vi "llh2lcctmp.vi"(7 "map name":T1(ring)=enum."KAIST", 9 "hgt[deg]":i32, 10 "lon[deg]":dbl format="%#_12f", 11 "lat[deg]":dbl format="%#_12f") -> (3 "LCC[m]":dbl[](array[numeric]))   [LabVIEW 2015]
uses:
  <vilib>/Analysis/Matrix/Numeric/Conversions/Array To Matrix - RA2.vi
  <vilib>/Analysis/Matrix/Numeric/Conversions/Array To Matrix - RA.vi
  <vilib>/Analysis/Matrix/Numeric/Multiply/Multiply - RM,RM.vi
  <vilib>/Analysis/Matrix/Numeric/Conversions/Matrix To Array - RM.vi
  <vilib>/Analysis/Matrix/NI_Matrix.lvlib
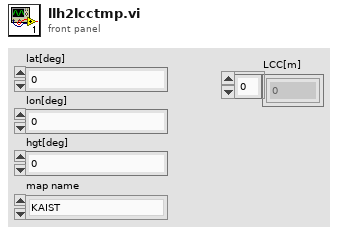
[diagram p1: front panel]
types:
  T1 = enum32{"Namyang", "Hyundai", "KAIST", "Ajou", "Munji", "Airforce", "Car", "KATRI", "Samsung", "Coex", "Gwangnaru", "Inje", "sinjin"}
  T2 = typedef "NI_Matrix.lvlib/RealMatrix.ctl" = dbl[][]
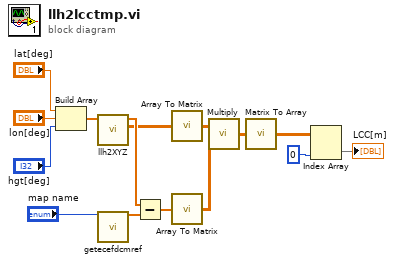
[diagram p0: block diagram]
diagram:
  n1 = Build Array("lat[deg]", "lon[deg]", "hgt[deg]") -> (w15:dbl[])
  n2 = call "llh2XYZ.vi"("llh"=w15) -> ("DCM(ecef2lcc)"=w4:dbl[][], "ecef"=w5:dbl[])  [unwired: 7 in]
  n3 = call "getecefdcmref.vi"("map name"="map name") -> ("XYZ"=w2:dbl[])  [unwired: 10 in, 4 out]
  n4 = Subtract(x=w5, y=w2) -> (x-y=w10:dbl[])
  n5 = call-poly <vilib>:"Array To Matrix.vi"("Real 2D Array"=w4) -> ("Real Matrix"=w11:T2)
  n6 = call-poly <vilib>:"Array To Matrix.vi"("Real 1D Array"=w10) -> ("Real Matrix (Column Vector)"=w9:T2)
  n7 = call-poly <vilib>:"Multiply.vi"("Real Matrix B"=w9, "Real Matrix A"=w11) -> ("A * B"=w8:T2)
  n8 = call-poly <vilib>:"Matrix To Array.vi"("Real Matrix"=w8) -> ("Real 2D Array"=w7:dbl[][])
  n9 = Index Array(array=w7, index (col)=0 ("disabled index (col)")) -> (element=→"LCC[m]":dbl[])  [unwired: 1 in]
